vi "BLE v1.0.vi"(7 "Est Thresh Val":dbl, 8 "Threshold Value Analysis":bool, 9 "Model Name":string="and_RB_SSA", 10 "Ex_Mod_IDs":string[](array[string]), 11 "Sp_Id_Arr":string[](array[string])) -> (0 "Close 2":bool, 3 "Boolean  Expression":string)   [LabVIEW 2014]
uses:
  <vilib>/Utility/file.llb/Read From Spreadsheet File (DBL).vi
  <vilib>/Utility/file.llb/Read From Spreadsheet File (string).vi
panel:
  out "Input Status":bool
  out "% fitness":string
  out "Row header":string[](array[string])
  out "Simulation Data":string[][](table)
  in  "Close":bool
  out "No of I/ps":i32
  out "Thresh Val":dbl[](array[numeric])
  out "All Data":string[][](array[string])
  out "Analog Data":dbl[][](array[numeric])
  out "All Data":dbl[][](array[numeric])
  out "Index":i32[](array[numeric])
  out "C1_Ar":dbl[](array[numeric])
  out "C2_Ar":dbl[](array[numeric])
  out "C3_Ar":dbl[](array[numeric])
  out "C4_Ar":dbl[](array[numeric])
  out "Cs4_1s":i32
  out "Cs3_1s":i32
  out "Cs2_1s":i32
  out "Cs1_1s":i32
  out "var_4":i8
  out "var_3":i8
  out "var_2":i8
  out "var_1":i8
  out "case4":i32
  out "case3":i32
  out "case2":i32
  out "case1":i32
  out "C4":dbl
  out "C3":dbl
  out "C2":dbl
  out "C1":dbl
  out "Digital Data":bool[][](array[boolean])
  # "Logic Expression"
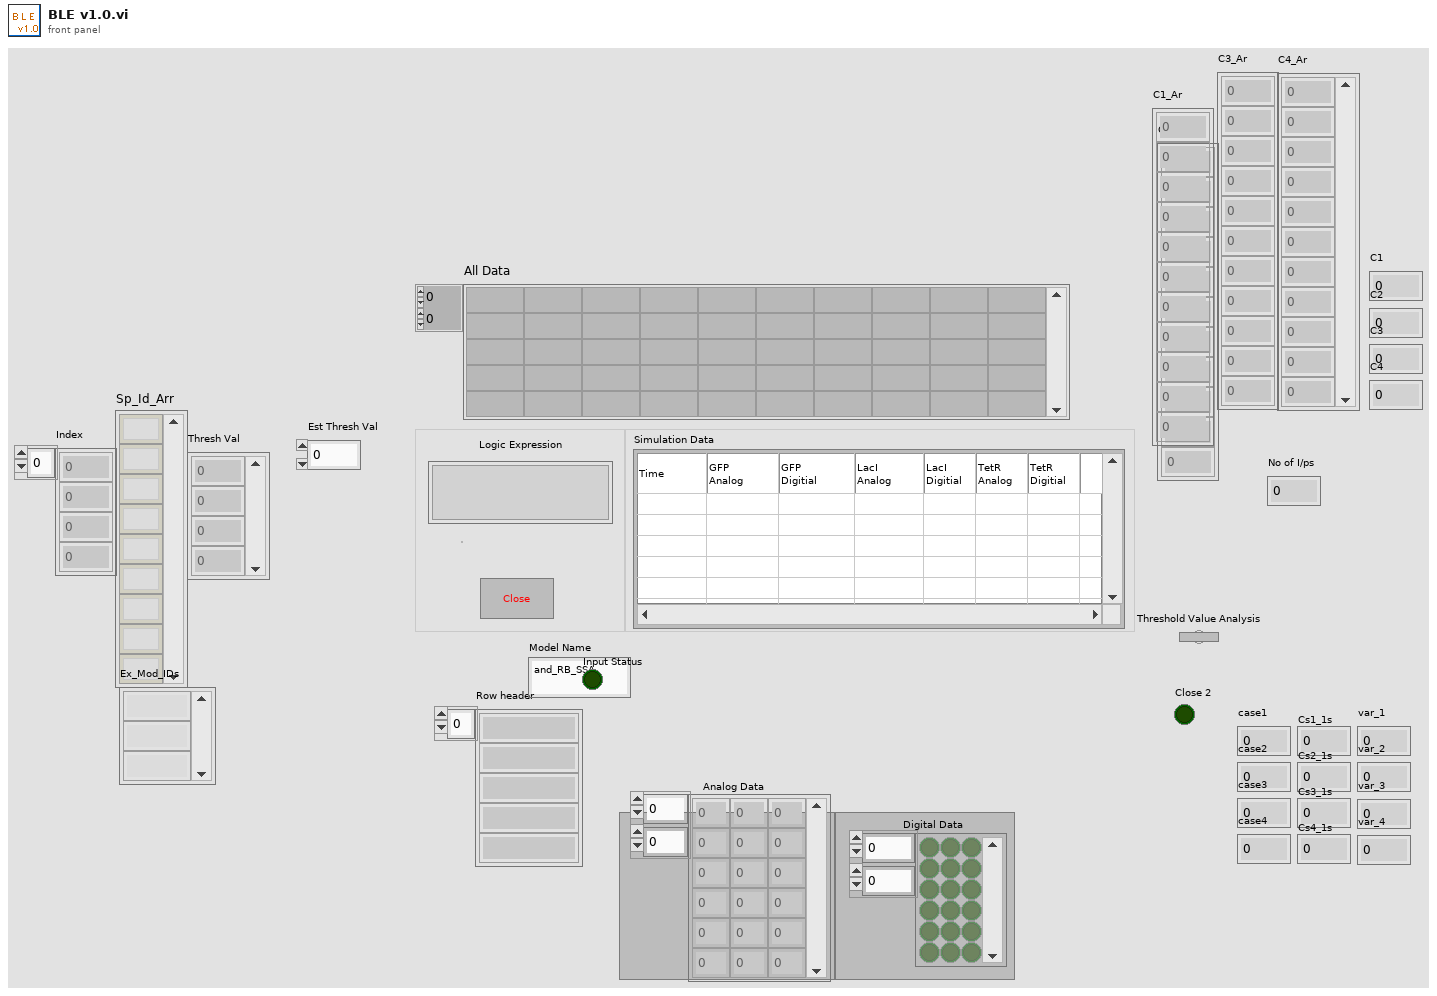
[diagram p1: front panel]
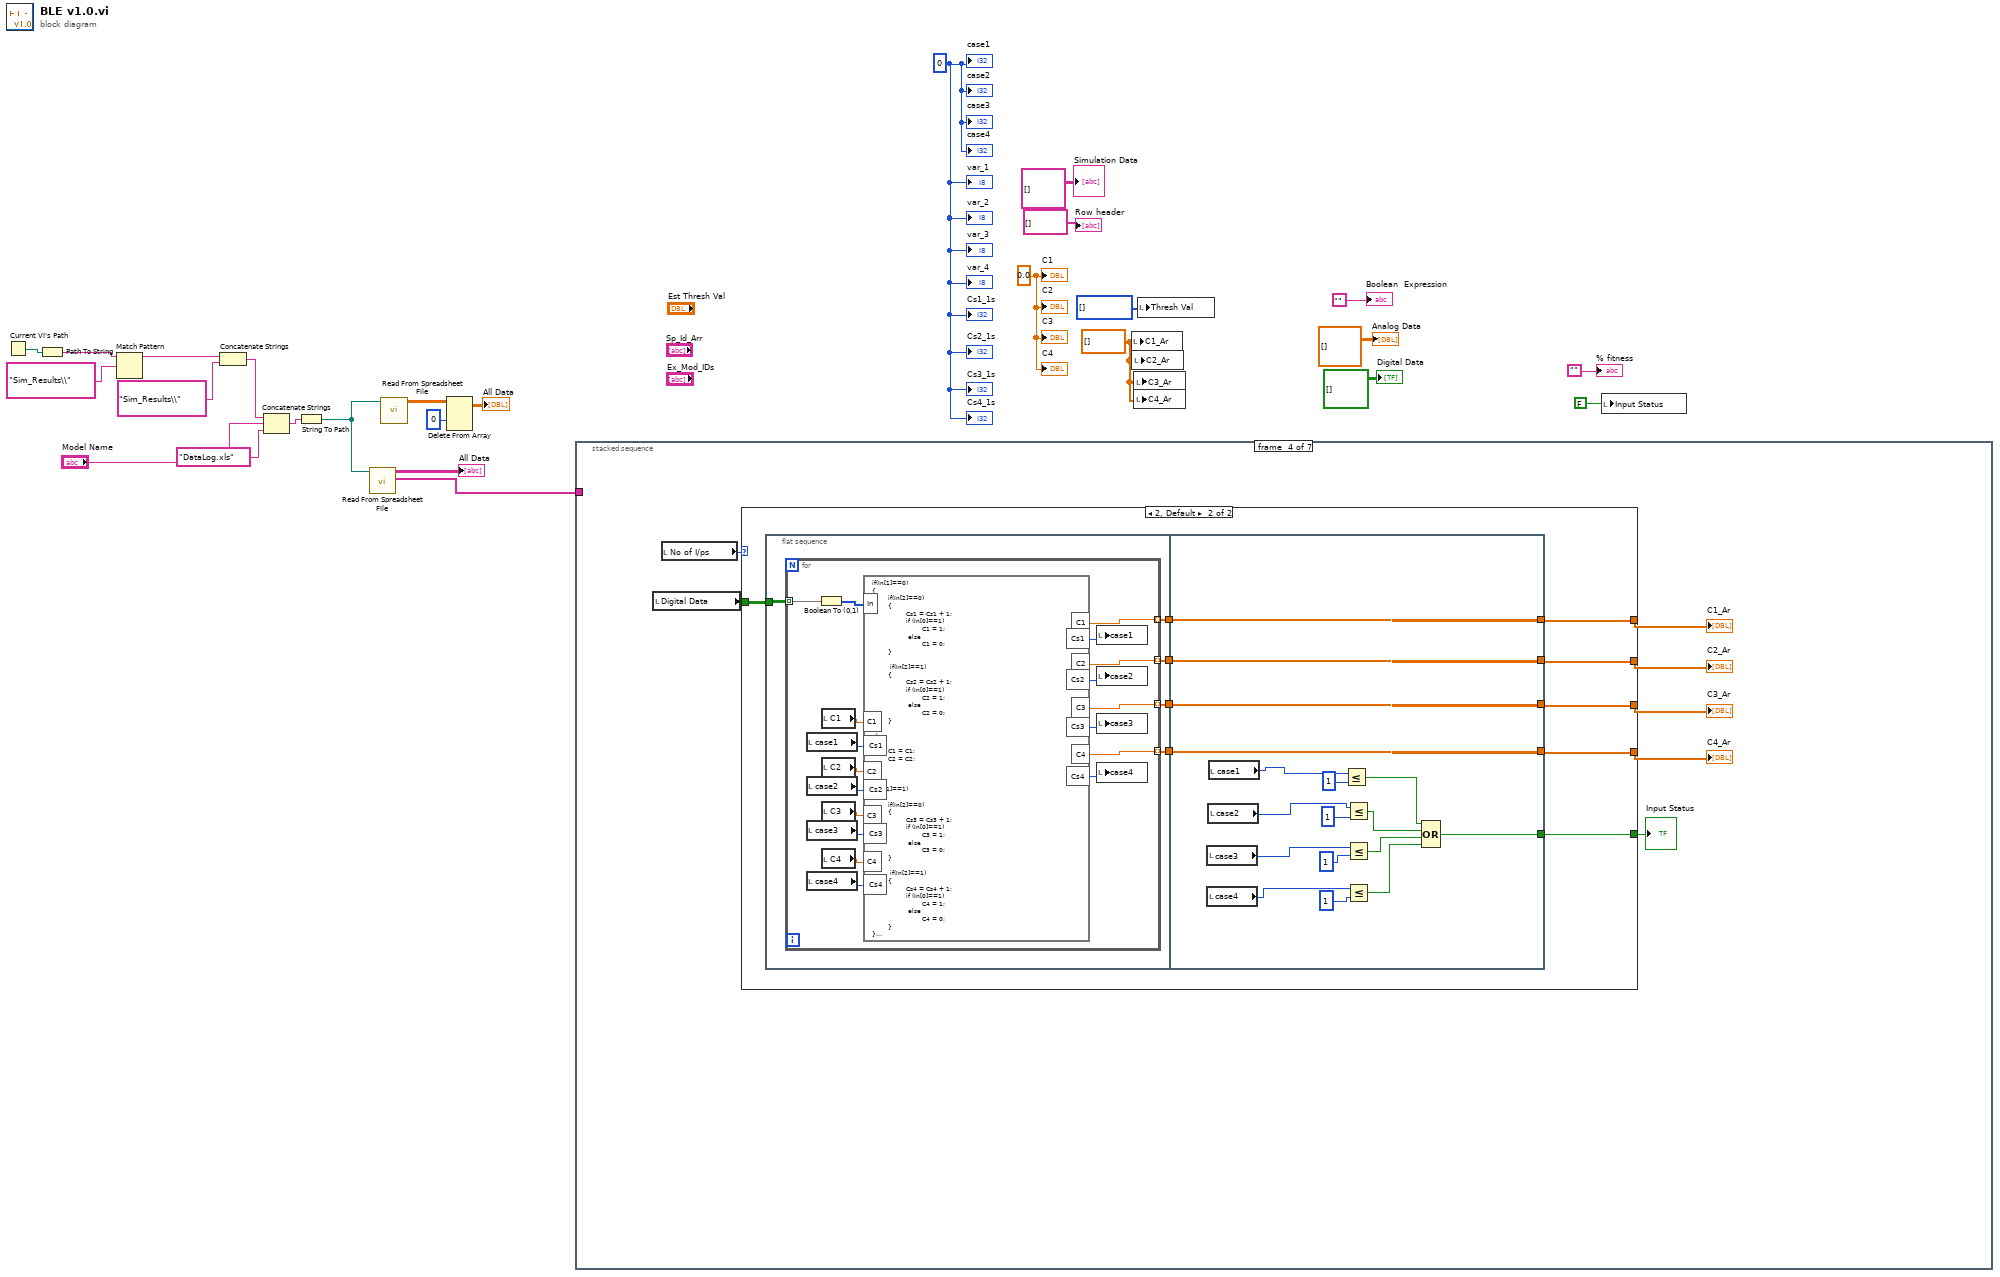
[diagram p0: block diagram]
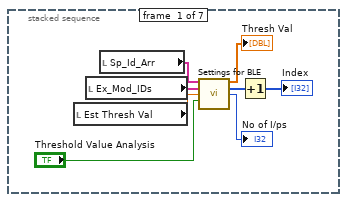
[diagram p2: hidden frame]
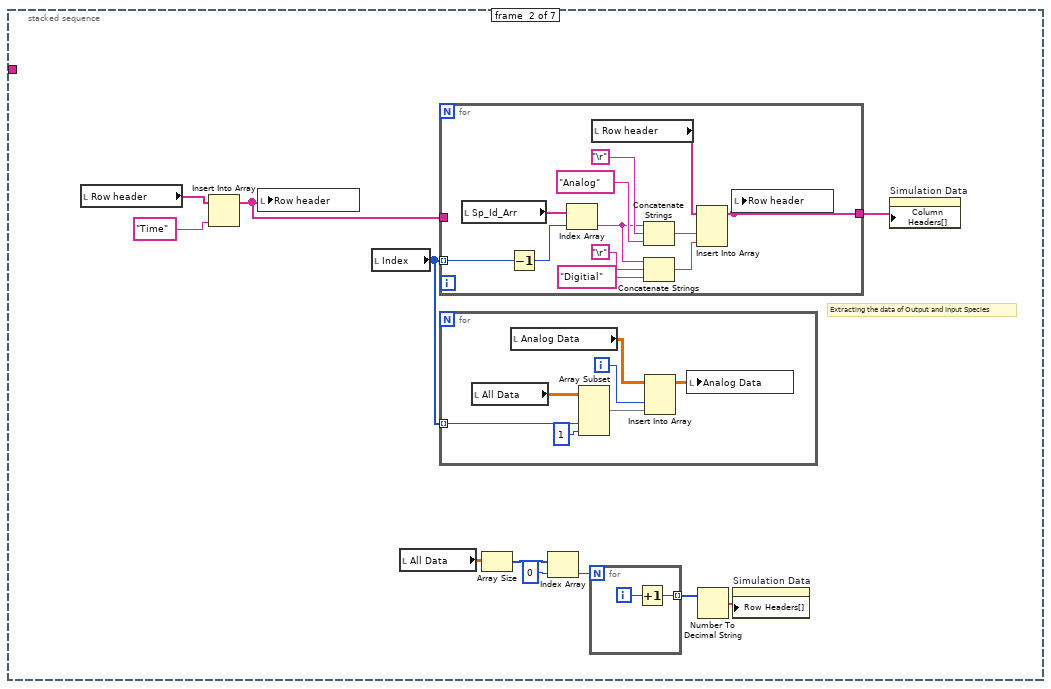
[diagram p3: hidden frame]
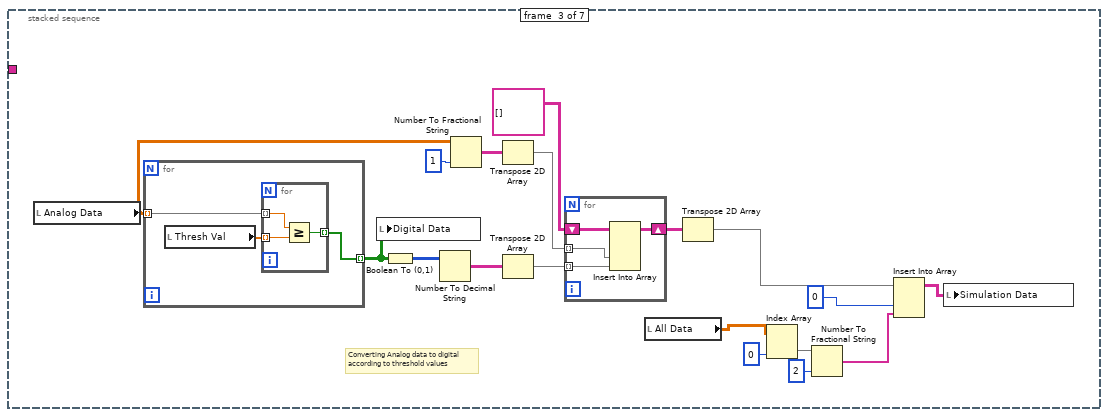
[diagram p4: hidden frame]
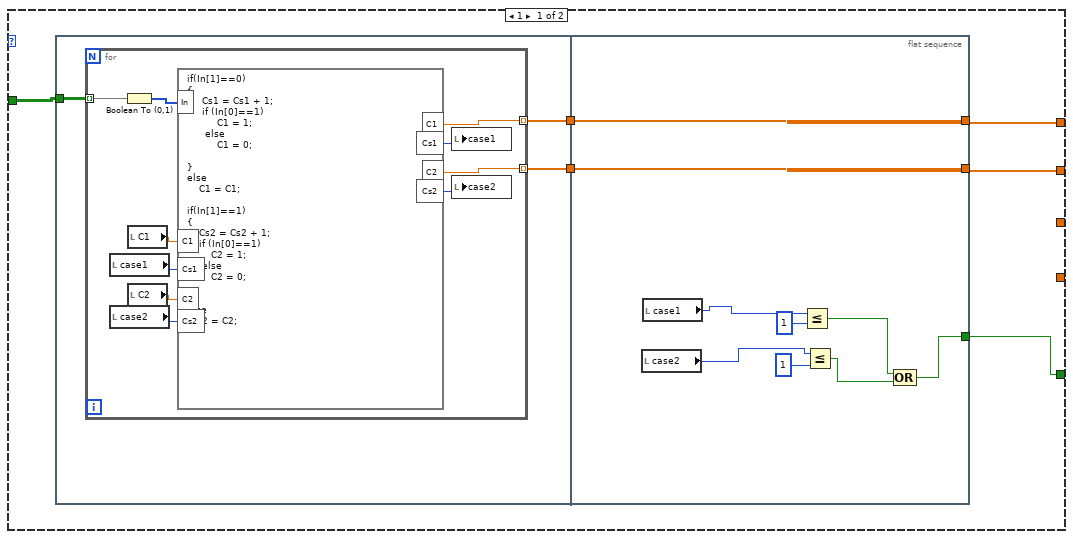
[diagram p5: hidden frame]
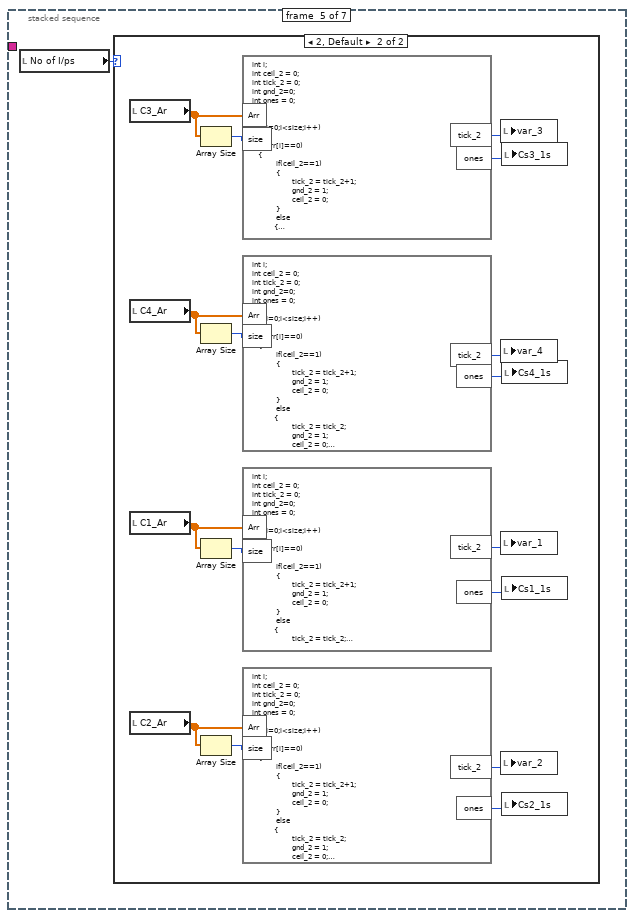
[diagram p6: hidden frame]
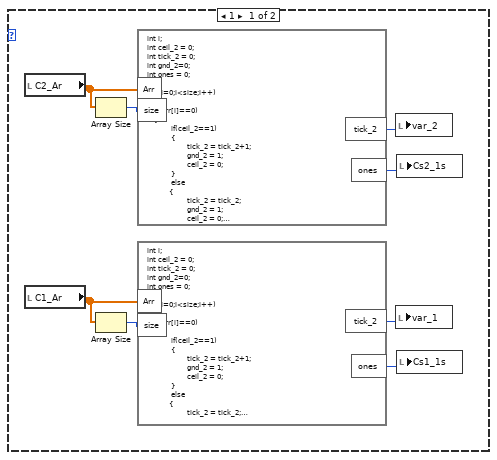
[diagram p7: hidden frame]
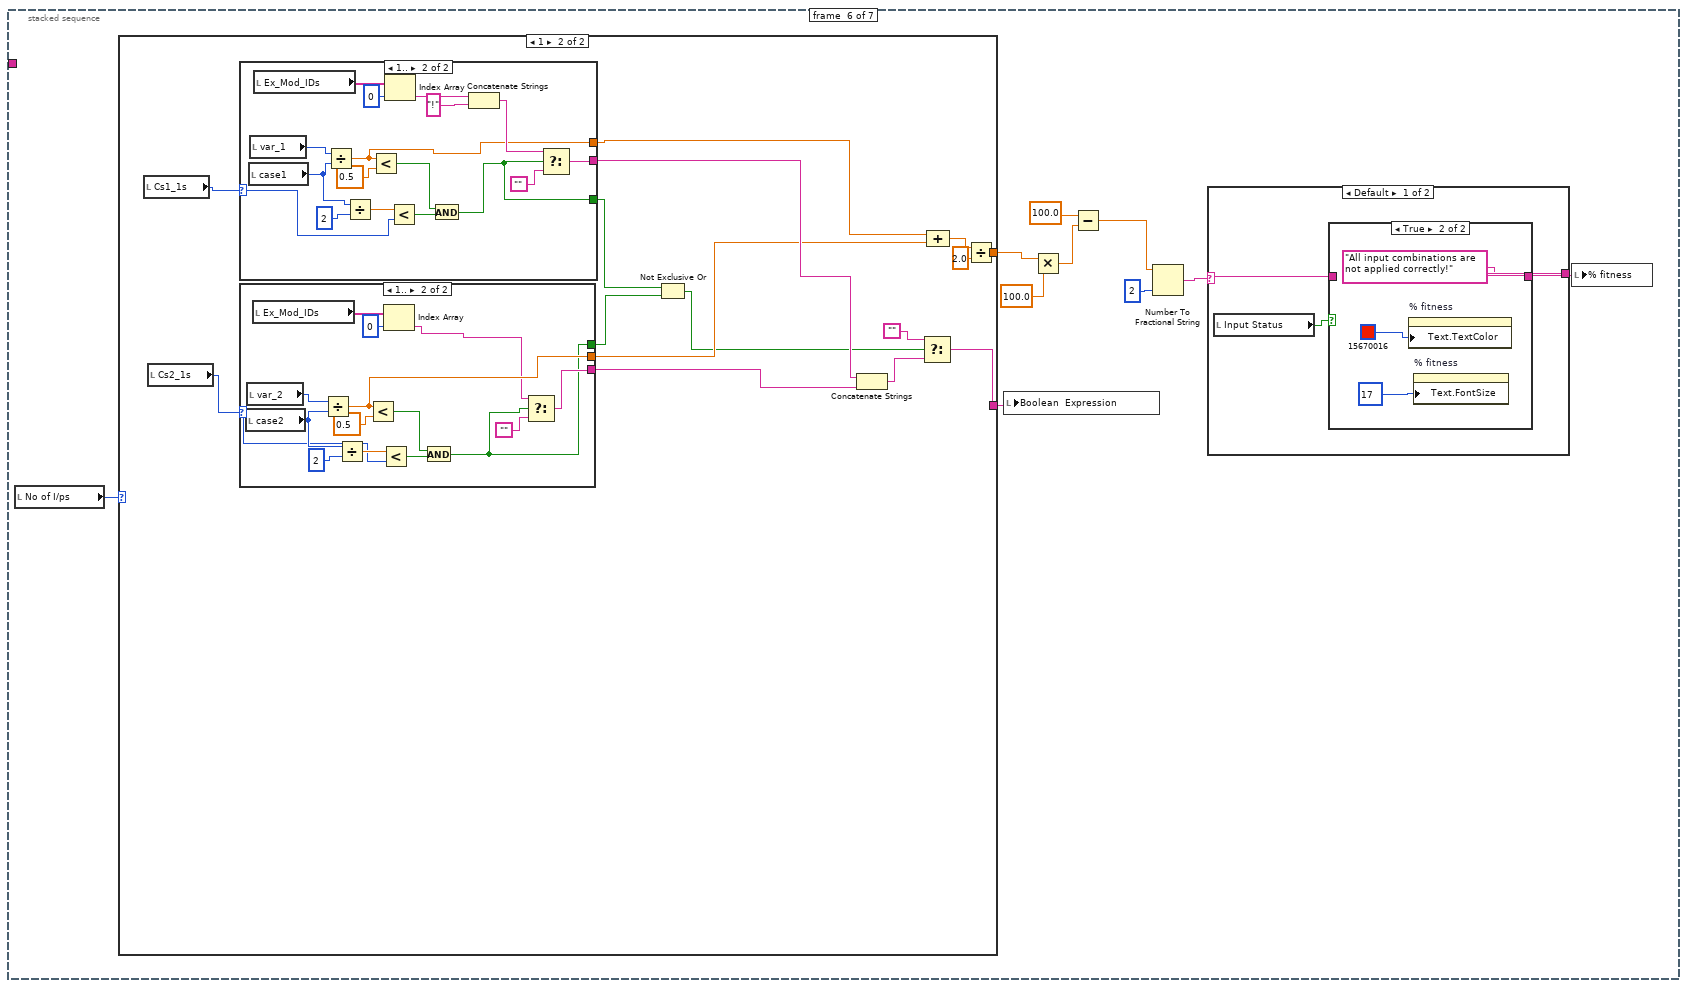
[diagram p8: hidden frame]
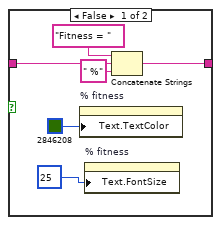
[diagram p9: hidden frame]
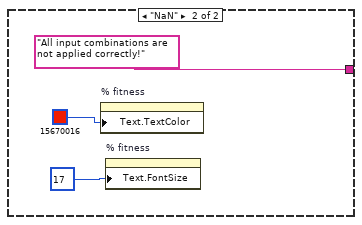
[diagram p10: hidden frame]
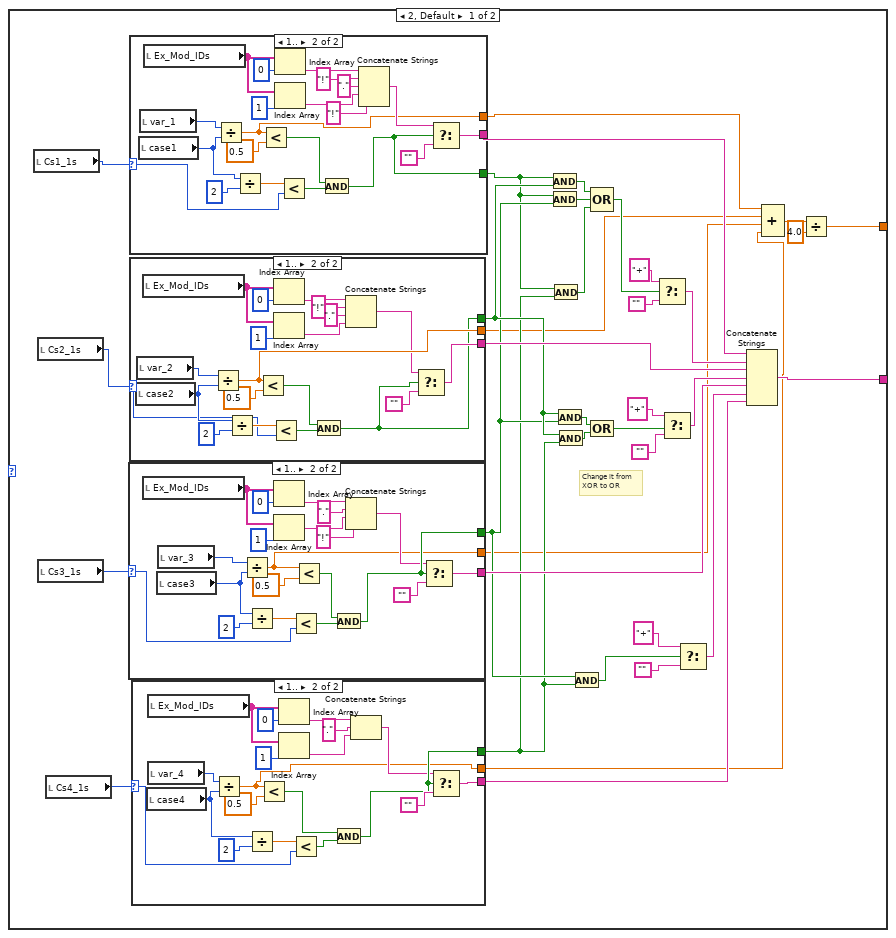
[diagram p11: hidden frame]
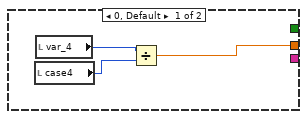
[diagram p12: hidden frame]
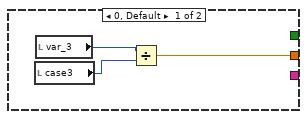
[diagram p13: hidden frame]
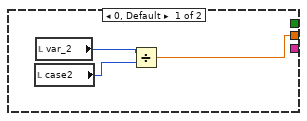
[diagram p14: hidden frame]
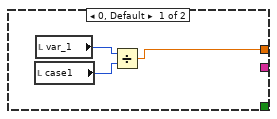
[diagram p15: hidden frame]
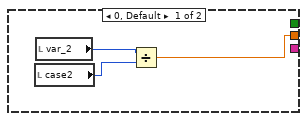
[diagram p16: hidden frame]
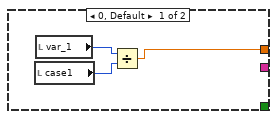
[diagram p17: hidden frame]
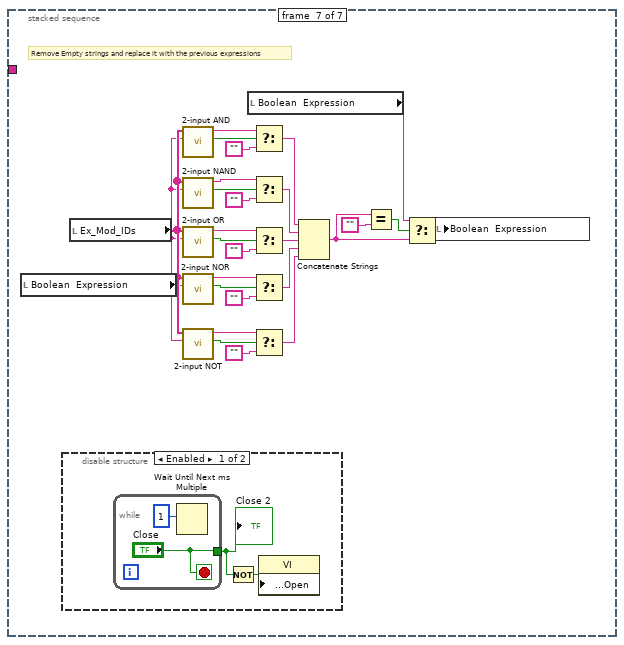
[diagram p18: hidden frame]
diagram:
  w21 = 0.0 ("C1")
  w22 = 0 ("case1")
  w26 = dbl[] [] ("C1_Ar")
  n1 = Current VI's Path() -> (path=w6:path)
  n2 = Path To String(path=w6) -> (string=w7:string)
  n3 = Match Pattern(string=w7, regular expression="Sim_Results\\" ("string")) -> (before substring=w9:string)  [unwired: 1 in, 3 out]
  n4 = Concatenate Strings(w9, "Sim_Results\\" ("string")) -> (w5:string)
  n5 = Concatenate Strings(w5, "Model Name", "DataLog.xls" ("name or relative path")) -> (w4:string)
  n6 = String To Path(string=w4) -> (path=w3:path)
  n7 = call-poly <vilib>:"Read From Spreadsheet File.vi"("file path (dialog if empty)"=w3) -> ("first row"=w13:string[], "all rows"=→"All Data":string[][])  [unwired: 6 in, 3 out]
  n8 = call-poly <vilib>:"Read From Spreadsheet File.vi"("file path (dialog if empty)"=w3) -> ("all rows"=w16:dbl[][])  [unwired: 6 in, 4 out]
  n9 = Delete From Array(array=w16, index (row)=0) -> (array with subset deleted=→"All Data":dbl[][])  [unwired: 2 in, 1 out]
  n10 = stacked-sequence {
    tunnel: w13 -> [_ _ _ _ _ _ _]
    frame #0 {
      n11 = local read "Est Thresh Val"() -> (w27:dbl)
      n12 = local read "Ex_Mod_IDs"() -> (w33:string[])
      n13 = local read "Sp_Id_Arr"() -> (w34:string[])
      n14 = call "Settings for BLE.vi"("Sp_Id_Arr"=w34, "Ex_Mod_IDs"=w33, "Est Thresh Val"=w27, "Threshold Value Analysis"="Threshold Value Analysis") -> ("Thresh Val"=→"Thresh Val":dbl[], "Index"=w31:i32[], "No of I/ps"=→"No of I/ps":i32)  [unwired: 9 in]
      n15 = Increment(x=w31) -> (x+1=→"Index":i32[])
    }
    frame #1 {
      # "Extracting the data of Output and Input Species"
      n16 = local read "Row header"() -> (w37:string[])
      n17 = Insert Into Array(array=w37, new element="Time" ("new element/subarray")) -> (w35:string[])  [unwired: 1 in]
      n18 = local write "Row header"(w35) -> ()
      n19 = local read "Index"() -> (w45:i32[])
      n20 = local read "All Data"() -> (w43:dbl[][])
      n21 = for {
        tunnel: w45 -> [w58] mode=indexing
        tunnel: [w49] -> w44
        tunnel: w35 -> [_]
        n22 = local read "Sp_Id_Arr"() -> (w59:string[])
        n23 = Decrement(x=w58) -> (x-1=w57:i32)
        n24 = Index Array(array=w59, index=w57) -> (element=w51:string)
        n25 = local read "Row header"() -> (w48:string[])
        n26 = Concatenate Strings(w51, "\r", "Analog" ("string")) -> (w54:string)
        n27 = Concatenate Strings(w51, "\r", "Digitial" ("string")) -> (w50:string)
        n28 = Insert Into Array(array=w48, new element #1=w54, new element #2=w50) -> (w49:string[])  [unwired: 1 in]
        n29 = local write "Row header"(w49) -> ()
      }
      n30 = for {
        tunnel: w45 -> [w65] mode=indexing
        i -> [w62]
        n31 = local read "All Data"() -> (w66:dbl[][])
        n32 = local read "Analog Data"() -> (w61:dbl[][])
        n33 = Array Subset(array=w66, index (col)=w65, length (col)=1 ("length")) -> (w63:dbl[][])  [unwired: 2 in]
        n34 = Insert Into Array(array=w61, index (col)=w62, new element=w63) -> (w60:dbl[][])  [unwired: 1 in]
        n35 = local write "Analog Data"(w60) -> ()
      }
      n36 = Array Size(array=w43) -> (size(s)=w42:i32[])
      n37 = Index Array(array=w42, index=0) -> (element=w40:i32)
      n38 = for {
        N: w40 -> [_]
        tunnel: [w46] -> w39 mode=indexing
        i -> [w47]
        n39 = Increment(x=w47) -> (x+1=w46:i32)
      }
      n40 = Number To Decimal String(number=w39) -> (decimal integer string=w38:string[])  [unwired: 1 in]
      n41 = property on="Simulation Data" class="Tbl (strict)"("Row Headers[]"=w38) -> ()  [unwired: 2 in, 2 out]
      n42 = property on="Simulation Data" class="Tbl (strict)"("Column Headers[]"=w44) -> ()  [unwired: 2 in, 2 out]
    }
    frame #2 {
      # "Converting Analog data to digital\naccording to threshold values"
      n43 = local read "Analog Data"() -> (w80:dbl[][])
      n44 = for {
        tunnel: w80 -> [w90] mode=indexing
        tunnel: [w89] -> w82 mode=indexing
        n45 = local read "Thresh Val"() -> (w91:dbl[])
        n46 = for {
          tunnel: w90 -> [w93] mode=indexing
          tunnel: w91 -> [w94] mode=indexing
          tunnel: [w92] -> w89 mode=indexing
          n47 = Greater Or Equal?(x=w93, y=w94) -> (x >= y?=w92:bool)
        }
      }
      n48 = local write "Digital Data"(w82) -> ()
      n49 = Boolean To (0,1)(Boolean=w82) -> (0, 1=w83:i16[][])
      n50 = Number To Decimal String(number=w83) -> (decimal integer string=w77:string[][])  [unwired: 1 in]
      n51 = Number To Fractional String(number=w80, precision (6)=i16 1) -> (F-format string=w79:string[][])  [unwired: 2 in]
      n52 = Transpose 2D Array(2D array=w79) -> (transposed array=w78:string[][])
      n53 = Transpose 2D Array(2D array=w77) -> (transposed array=w76:string[][])
      n54 = for {
        shift-right: [w88] -> w75
        shift-left: string[][] [] -> [w87]
        tunnel: w76 -> [w86] mode=indexing
        tunnel: w78 -> [w85] mode=indexing
        n55 = Insert Into Array(array=w87, new element #1=w85, new element #2=w86) -> (w88:string[][])  [unwired: 2 in]
      }
      n56 = local read "All Data"() -> (w68:dbl[][])
      n57 = Transpose 2D Array(2D array=w75) -> (transposed array=w69:string[][])
      n58 = Index Array(array=w68, index (col)=0 ("disabled index (col)")) -> (element=w71:dbl[])  [unwired: 1 in]
      n59 = Number To Fractional String(number=w71, precision (6)=i16 2) -> (F-format string=w73:string[])  [unwired: 2 in]
      n60 = Insert Into Array(array=w69, index (col)=0 ("disabled index (col)"), new element=w73) -> (w67:string[][])  [unwired: 1 in]
      n61 = local write "Simulation Data"(w67) -> ()
    }
    frame #3 {
      n62 = local read "Digital Data"() -> (w101:bool[][])
      n63 = local read "No of I/ps"() -> (w96:i32)
      n64 = case shown="2, Default" w96 {
        tunnel: w101 -> [w107 w139]
        tunnel: [w105 w138] -> w100
        tunnel: [w106 w137] -> w99
        tunnel: [_ w136] -> w98
        tunnel: [_ w135] -> w97
        tunnel: [w102 w130] -> w95
        frame 1 {
          n65 = flat-sequence {
            tunnel: w107 -> [w110]
            tunnel: [w109] -> w104
            tunnel: [w108] -> w103
            tunnel: [w128] -> w105
            tunnel: [w129] -> w106
            tunnel: w104 -> [w129]
            tunnel: w103 -> [w128]
            tunnel: [w121] -> w102
            frame #0 {
              n66 = for {
                tunnel: [w113] -> w108 mode=indexing
                tunnel: [w112] -> w109 mode=indexing
                tunnel: w110 -> [w111] mode=indexing
                n67 = local read "case1"() -> (w118:i32)
                n68 = local read "case2"() -> (w117:i32)
                n69 = Boolean To (0,1)(Boolean=w111) -> (0, 1=w120:i16[])
                n70 = local read "C1"() -> (w116:dbl)
                n71 = local read "C2"() -> (w119:dbl)
                n72 = formula code="if(In[1]==0)\n{\n     Cs1 = Cs1 + 1;\n     if (In[0]==1)\n          C1 = 1;\n      else\n          C1 = 0;\n\n}\nelse\n    C1 = C1;\n\nif(In[1]==1)\n{\n    Cs2 = Cs2 + 1;\n    if (In[0]==1)\n        C2 = 1;\n     else\n        C2 = 0;\n\n}\nelse\n   C2 = C2;"("In"=w120, "C1"=w116, "C2"=w119, "Cs1"=w118, "Cs2"=w117) -> ("C1"=w113:dbl, "C2"=w112:dbl, "Cs1"=w114:i32, "Cs2"=w115:i32)
                n73 = local write "case1"(w114) -> ()
                n74 = local write "case2"(w115) -> ()
              }
            }
            frame #1 {
              n75 = local read "case2"() -> (w122:i32)
              n76 = local read "case1"() -> (w123:i32)
              n77 = Less Or Equal?(x=w123, y=1) -> (x <= y?=w125:bool)
              n78 = Less Or Equal?(x=w122, y=1) -> (x <= y?=w124:bool)
              n79 = Compound Arithmetic op=OR(w125, w124) -> (w121:bool)
            }
          }
        }
        frame 2, Default {
          n80 = flat-sequence {
            tunnel: w139 -> [w144]
            tunnel: [w143] -> w134
            tunnel: [w142] -> w133
            tunnel: [w141] -> w132
            tunnel: [w140] -> w131
            tunnel: [w176] -> w135
            tunnel: [w177] -> w136
            tunnel: [w178] -> w137
            tunnel: [w179] -> w138
            tunnel: w134 -> [w179]
            tunnel: w133 -> [w178]
            tunnel: w132 -> [w177]
            tunnel: w131 -> [w176]
            tunnel: [w163] -> w130
            frame #0 {
              n81 = for {
                tunnel: w144 -> [w162] mode=indexing
                tunnel: [w148] -> w143 mode=indexing
                tunnel: [w147] -> w142 mode=indexing
                tunnel: [w146] -> w141 mode=indexing
                tunnel: [w145] -> w140 mode=indexing
                n82 = local read "case1"() -> (w157:i32)
                n83 = local read "case2"() -> (w154:i32)
                n84 = local read "case3"() -> (w156:i32)
                n85 = local read "case4"() -> (w155:i32)
                n86 = Boolean To (0,1)(Boolean=w162) -> (0, 1=w161:i16[])
                n87 = local read "C1"() -> (w153:dbl)
                n88 = local read "C2"() -> (w160:dbl)
                n89 = local read "C3"() -> (w159:dbl)
                n90 = local read "C4"() -> (w158:dbl)
                n91 = formula code="if(In[1]==0)\n{\n        if(In[2]==0)\n        {\n                 Cs1 = Cs1 + 1;\n                 if (In[0]==1)\n                         C1 = 1;\n                  else\n                         C1 = 0;\n        }\n\n         if(In[2]==1)\n        {\n                 Cs2 = Cs2 + 1;\n                 if (In[0]==1)\n                         C2 = 1;\n                  else\n                         C2 = 0;\n        }  \n}\nelse\n{\n        C1 = C1;\n        C2 = C2;\n}\n\n\nif(In[1]==1)\n{\n        if(In[2]==0)\n        {\n                 Cs3 = Cs3 + 1;\n                 if (In[0]==1)\n                         C3 = 1;\n                  else\n                         C3 = 0;\n        }\n\n         if(In[2]==1)\n        {\n                 Cs4 = Cs4 + 1;\n                 if (In[0]==1)\n                         C4 = 1;\n                  else\n                         C4 = 0;\n        }  \n}\nelse\n{\n        C3 = C3;\n        C4 = C4;\n}"("In"=w161, "C1"=w153, "C2"=w160, "C3"=w159, "C4"=w158, "Cs1"=w157, "Cs2"=w154, "Cs3"=w156, "Cs4"=w155) -> ("C1"=w148:dbl, "C2"=w147:dbl, "C3"=w146:dbl, "C4"=w145:dbl, "Cs1"=w149:i32, "Cs2"=w150:i32, "Cs3"=w151:i32, "Cs4"=w152:i32)
                n92 = local write "case1"(w149) -> ()
                n93 = local write "case2"(w150) -> ()
                n94 = local write "case3"(w151) -> ()
                n95 = local write "case4"(w152) -> ()
              }
            }
            frame #1 {
              n96 = local read "case3"() -> (w165:i32)
              n97 = local read "case4"() -> (w164:i32)
              n98 = local read "case2"() -> (w166:i32)
              n99 = local read "case1"() -> (w167:i32)
              n100 = Less Or Equal?(x=w167, y=1) -> (x <= y?=w171:bool)
              n101 = Less Or Equal?(x=w166, y=1) -> (x <= y?=w170:bool)
              n102 = Less Or Equal?(x=w165, y=1) -> (x <= y?=w169:bool)
              n103 = Less Or Equal?(x=w164, y=1) -> (x <= y?=w168:bool)
              n104 = Compound Arithmetic op=OR(w171, w170, w169, w168) -> (w163:bool)
            }
          }
        }
      }
      "C1_Ar" <- w100
      "C2_Ar" <- w99
      "C3_Ar" <- w98
      "C4_Ar" <- w97
      "Input Status" <- w95
    }
    frame #4 {
      n105 = local read "No of I/ps"() -> (w180:i32)
      n106 = case shown="2, Default" w180 {
        frame 1 {
          n107 = local read "C2_Ar"() -> (w185:dbl[])
          n108 = local read "C1_Ar"() -> (w186:dbl[])
          n109 = Array Size(array=w185) -> (size(s)=w187:i32)
          n110 = Array Size(array=w186) -> (size(s)=w188:i32)
          n111 = formula code="int i;\nint ceil_2 = 0;\nint tick_2 = 0;\nint gnd_2=0;\nint ones = 0;\n\nfor (i=0;i<size;i++)\n{\n   if(Arr[i]==0)\n   { \n            if(ceil_2==1)\n            {\n                    tick_2 = tick_2+1;\n                    gnd_2 = 1;\n                    ceil_2 = 0;\n            }\n            else \n           {\n                    tick_2 = tick_2;\n                    gnd_2 = 1;\n                    ceil_2 = 0;                 \n           } \n   }\n   \n   else if(Arr[i]==1)\n   {\n            ones = ones +1;\n            if(gnd_2==1)\n            {\n                    tick_2 = tick_2+1;\n                    gnd_2 = 0;\n                    ceil_2 = 1;\n            }\n            else \n           {\n                    tick_2 = tick_2;\n                    gnd_2 = gnd_2;\n                    ceil_2 = 1;                 \n           } \n   }\n   else\n   {\n           tick_2 = tick_2;\n           ceil_2 = ceil_2;\n           gnd_2 = gnd_2;\n   }\n}"("Arr"=w185, "size"=w187) -> ("tick_2"=w182:i32, "ones"=w181:i32)
          n112 = formula code="int i;\nint ceil_2 = 0;\nint tick_2 = 0;\nint gnd_2=0;\nint ones = 0;\n\nfor (i=0;i<size;i++)\n{\n   if(Arr[i]==0)\n   { \n            if(ceil_2==1)\n            {\n                    tick_2 = tick_2+1;\n                    gnd_2 = 1;\n                    ceil_2 = 0;\n            }\n            else \n           {\n                    tick_2 = tick_2;\n                    gnd_2 = 1;\n                    ceil_2 = 0;                 \n           } \n   }\n   \n   else if(Arr[i]==1)\n   {\n            ones = ones +1;\n            if(gnd_2==1)\n            {\n                    tick_2 = tick_2+1;\n                    gnd_2 = 0;\n                    ceil_2 = 1;\n            }\n            else \n           {\n                    tick_2 = tick_2;\n                    gnd_2 = gnd_2;\n                    ceil_2 = 1;                 \n           } \n   }\n   else\n   {\n           tick_2 = tick_2;\n           ceil_2 = ceil_2;\n           gnd_2 = gnd_2;\n   }\n}"("Arr"=w186, "size"=w188) -> ("tick_2"=w184:i32, "ones"=w183:i32)
          n113 = local write "var_2"(w182) -> ()
          n114 = local write "var_1"(w184) -> ()
          n115 = local write "Cs2_1s"(w181) -> ()
          n116 = local write "Cs1_1s"(w183) -> ()
        }
        frame 2, Default {
          n117 = local read "C3_Ar"() -> (w197:dbl[])
          n118 = local read "C4_Ar"() -> (w199:dbl[])
          n119 = local read "C1_Ar"() -> (w200:dbl[])
          n120 = local read "C2_Ar"() -> (w198:dbl[])
          n121 = Array Size(array=w197) -> (size(s)=w203:i32)
          n122 = Array Size(array=w199) -> (size(s)=w201:i32)
          n123 = Array Size(array=w200) -> (size(s)=w204:i32)
          n124 = Array Size(array=w198) -> (size(s)=w202:i32)
          n125 = formula code="int i;\nint ceil_2 = 0;\nint tick_2 = 0;\nint gnd_2=0;\nint ones = 0;\n\n\nfor (i=0;i<size;i++)\n{\n   if(Arr[i]==0)\n   { \n            if(ceil_2==1)\n            {\n                    tick_2 = tick_2+1;\n                    gnd_2 = 1;\n                    ceil_2 = 0;\n            }\n            else \n           {\n                    tick_2 = tick_2;\n                    gnd_2 = 1;\n                    ceil_2 = 0;                 \n           } \n   }\n   \n   else if(Arr[i]==1)\n   {\n            ones = ones +1;\n            if(gnd_2==1)\n            {\n                    tick_2 = tick_2+1;\n                    gnd_2 = 0;\n                    ceil_2 = 1;\n            }\n            else \n           {\n                    tick_2 = tick_2;\n                    gnd_2 = gnd_2;\n                    ceil_2 = 1;                 \n           } \n   }\n   else\n   {\n           tick_2 = tick_2;\n           ceil_2 = ceil_2;\n           gnd_2 = gnd_2;\n   }\n}"("Arr"=w197, "size"=w203) -> ("tick_2"=w192:i32, "ones"=w191:i32)
          n126 = formula code="int i;\nint ceil_2 = 0;\nint tick_2 = 0;\nint gnd_2=0;\nint ones = 0;\n\nfor (i=0;i<size;i++)\n{\n   if(Arr[i]==0)\n   { \n            if(ceil_2==1)\n            {\n                    tick_2 = tick_2+1;\n                    gnd_2 = 1;\n                    ceil_2 = 0;\n            }\n            else \n           {\n                    tick_2 = tick_2;\n                    gnd_2 = 1;\n                    ceil_2 = 0;                 \n           } \n   }\n   \n   else if(Arr[i]==1)\n   {\n            ones = ones +1;\n            if(gnd_2==1)\n            {\n                    tick_2 = tick_2+1;\n                    gnd_2 = 0;\n                    ceil_2 = 1;\n            }\n            else \n           {\n                    tick_2 = tick_2;\n                    gnd_2 = gnd_2;\n                    ceil_2 = 1;                 \n           } \n   }\n   else\n   {\n           tick_2 = tick_2;\n           ceil_2 = ceil_2;\n           gnd_2 = gnd_2;\n   }\n}"("Arr"=w199, "size"=w201) -> ("tick_2"=w190:i32, "ones"=w189:i32)
          n127 = formula code="int i;\nint ceil_2 = 0;\nint tick_2 = 0;\nint gnd_2=0;\nint ones = 0;\n\nfor (i=0;i<size;i++)\n{\n   if(Arr[i]==0)\n   { \n            if(ceil_2==1)\n            {\n                    tick_2 = tick_2+1;\n                    gnd_2 = 1;\n                    ceil_2 = 0;\n            }\n            else \n           {\n                    tick_2 = tick_2;\n                    gnd_2 = 1;\n                    ceil_2 = 0;                 \n           } \n   }\n   \n   else if(Arr[i]==1)\n   {\n            ones = ones +1;\n            if(gnd_2==1)\n            {\n                    tick_2 = tick_2+1;\n                    gnd_2 = 0;\n                    ceil_2 = 1;\n            }\n            else \n           {\n                    tick_2 = tick_2;\n                    gnd_2 = gnd_2;\n                    ceil_2 = 1;                 \n           } \n   }\n   else\n   {\n           tick_2 = tick_2;\n           ceil_2 = ceil_2;\n           gnd_2 = gnd_2;\n   }\n}"("Arr"=w200, "size"=w204) -> ("tick_2"=w196:i32, "ones"=w195:i32)
          n128 = formula code="int i;\nint ceil_2 = 0;\nint tick_2 = 0;\nint gnd_2=0;\nint ones = 0;\n\nfor (i=0;i<size;i++)\n{\n   if(Arr[i]==0)\n   { \n            if(ceil_2==1)\n            {\n                    tick_2 = tick_2+1;\n                    gnd_2 = 1;\n                    ceil_2 = 0;\n            }\n            else \n           {\n                    tick_2 = tick_2;\n                    gnd_2 = 1;\n                    ceil_2 = 0;                 \n           } \n   }\n   \n   else if(Arr[i]==1)\n   {\n            ones = ones +1;\n            if(gnd_2==1)\n            {\n                    tick_2 = tick_2+1;\n                    gnd_2 = 0;\n                    ceil_2 = 1;\n            }\n            else \n           {\n                    tick_2 = tick_2;\n                    gnd_2 = gnd_2;\n                    ceil_2 = 1;                 \n           } \n   }\n   else\n   {\n           tick_2 = tick_2;\n           ceil_2 = ceil_2;\n           gnd_2 = gnd_2;\n   }\n}"("Arr"=w198, "size"=w202) -> ("tick_2"=w194:i32, "ones"=w193:i32)
          n129 = local write "var_3"(w192) -> ()
          n130 = local write "var_4"(w190) -> ()
          n131 = local write "var_1"(w196) -> ()
          n132 = local write "var_2"(w194) -> ()
          n133 = local write "Cs3_1s"(w191) -> ()
          n134 = local write "Cs4_1s"(w189) -> ()
          n135 = local write "Cs1_1s"(w195) -> ()
          n136 = local write "Cs2_1s"(w193) -> ()
        }
      }
    }
    frame #5 {
      n137 = local read "No of I/ps"() -> (w211:i32)
      n138 = case shown="1" w211 {
        tunnel: [w249 w359] -> w214
        tunnel: [w230 w363] -> w212
        frame 2, Default {
          # "Change it from\nXOR to OR"
          n139 = local read "Cs1_1s"() -> (w266:i32)
          n140 = local read "Cs2_1s"() -> (w265:i32)
          n141 = local read "Cs3_1s"() -> (w264:i32)
          n142 = local read "Cs4_1s"() -> (w263:i32)
          n143 = case shown="1.." w264 {
            selector: w264 -> [_ w303]
            tunnel: [_ w301] -> w240
            tunnel: [_ w308] -> w252
            tunnel: [w289 w292] -> w234
            frame 0, Default {
              n144 = local read "case3"() -> (w291:i32)
              n145 = local read "var_3"() -> (w290:i8)
              n146 = Divide(x=w290, y=w291) -> (x/y=w289:dbl)
            }
            frame 1.. {
              n147 = local read "Ex_Mod_IDs"() -> (w295:string[])
              n148 = local read "case3"() -> (w304:i32)
              n149 = local read "var_3"() -> (w309:i8)
              n150 = Divide(x=w309, y=w304) -> (x/y=w292:dbl)
              n151 = Divide(x=w304, y=i8 2) -> (x/y=w307:dbl)
              n152 = Index Array(array=w295, index=0) -> (element=w298:string)
              n153 = Index Array(array=w295, index=1) -> (element=w296:string)
              n154 = Less?(x=w307, y=w303) -> (x < y?=w305:bool)
              n155 = Less?(x=w292, y=0.5) -> (x < y?=w302:bool)
              n156 = And(x=w302, y=w305) -> (x .and. y?=w301:bool)
              n157 = Concatenate Strings(w298, "." ("string"), w296, "!" ("string")) -> (w293:string)
              n158 = Select(t=w293, s=w301, f="") -> (s? t:f=w308:string)
            }
          }
          n159 = case shown="1.." w266 {
            selector: w266 -> [_ w350]
            tunnel: [_ w348] -> w237
            tunnel: [_ w355] -> w256
            tunnel: [w335 w338] -> w236
            frame 0, Default {
              n160 = local read "case1"() -> (w337:i32)
              n161 = local read "var_1"() -> (w336:i8)
              n162 = Divide(x=w336, y=w337) -> (x/y=w335:dbl)
            }
            frame 1.. {
              n163 = local read "case1"() -> (w351:i32)
              n164 = local read "var_1"() -> (w356:i8)
              n165 = local read "Ex_Mod_IDs"() -> (w339:string[])
              n166 = Divide(x=w356, y=w351) -> (x/y=w338:dbl)
              n167 = Divide(x=w351, y=i8 2) -> (x/y=w354:dbl)
              n168 = Less?(x=w338, y=0.5) -> (x < y?=w349:bool)
              n169 = Index Array(array=w339, index=0) -> (element=w345:string)
              n170 = Index Array(array=w339, index=1) -> (element=w342:string)
              n171 = Less?(x=w354, y=w350) -> (x < y?=w352:bool)
              n172 = And(x=w349, y=w352) -> (x .and. y?=w348:bool)
              n173 = Concatenate Strings(w345, "!" ("t"), "." ("string"), w342, "!" ("t")) -> (w340:string)
              n174 = Select(t=w340, s=w348, f="") -> (s? t:f=w355:string)
            }
          }
          n175 = case shown="1.." w265 {
            selector: w265 -> [_ w325]
            tunnel: [_ w323] -> w244
            tunnel: [_ w331] -> w254
            tunnel: [w312 w330] -> w235
            frame 0, Default {
              n176 = local read "case2"() -> (w313:i32)
              n177 = local read "var_2"() -> (w314:i8)
              n178 = Divide(x=w314, y=w313) -> (x/y=w312:dbl)
            }
            frame 1.. {
              n179 = local read "case2"() -> (w326:i32)
              n180 = local read "var_2"() -> (w332:i8)
              n181 = local read "Ex_Mod_IDs"() -> (w322:string[])
              n182 = Divide(x=w332, y=w326) -> (x/y=w330:dbl)
              n183 = Divide(x=w326, y=i8 2) -> (x/y=w327:dbl)
              n184 = Less?(x=w330, y=0.5) -> (x < y?=w324:bool)
              n185 = Less?(x=w327, y=w325) -> (x < y?=w329:bool)
              n186 = Index Array(array=w322, index=0) -> (element=w318:string)
              n187 = Index Array(array=w322, index=1) -> (element=w321:string)
              n188 = And(x=w324, y=w329) -> (x .and. y?=w323:bool)
              n189 = Concatenate Strings(w318, "!" ("t"), "." ("string"), w321) -> (w315:string)
              n190 = Select(t=w315, s=w323, f="") -> (s? t:f=w331:string)
            }
          }
          n191 = case shown="1.." w263 {
            selector: w263 -> [_ w281]
            tunnel: [_ w278] -> w239
            tunnel: [_ w285] -> w250
            tunnel: [w267 w270] -> w233
            frame 0, Default {
              n192 = local read "case4"() -> (w268:i32)
              n193 = local read "var_4"() -> (w269:i8)
              n194 = Divide(x=w269, y=w268) -> (x/y=w267:dbl)
            }
            frame 1.. {
              n195 = local read "case4"() -> (w280:i32)
              n196 = local read "Ex_Mod_IDs"() -> (w277:string[])
              n197 = local read "var_4"() -> (w286:i8)
              n198 = Divide(x=w286, y=w280) -> (x/y=w270:dbl)
              n199 = Divide(x=w280, y=i8 2) -> (x/y=w282:dbl)
              n200 = Less?(x=w270, y=0.5) -> (x < y?=w279:bool)
              n201 = Index Array(array=w277, index=0) -> (element=w274:string)
              n202 = Index Array(array=w277, index=1) -> (element=w276:string)
              n203 = Less?(x=w282, y=w281) -> (x < y?=w284:bool)
              n204 = And(x=w279, y=w284) -> (x .and. y?=w278:bool)
              n205 = Concatenate Strings(w274, "." ("string"), w276) -> (w271:string)
              n206 = Select(t=w271, s=w278, f="") -> (s? t:f=w285:string)
            }
          }
          n207 = And(x=w237, y=w244) -> (x .and. y?=w247:bool)
          n208 = And(x=w237, y=w240) -> (x .and. y?=w246:bool)
          n209 = And(x=w237, y=w239) -> (x .and. y?=w245:bool)
          n210 = And(x=w244, y=w240) -> (x .and. y?=w242:bool)
          n211 = And(x=w244, y=w239) -> (x .and. y?=w241:bool)
          n212 = And(x=w240, y=w239) -> (x .and. y?=w238:bool)
          n213 = Compound Arithmetic op=OR(w247, w246, w245) -> (w248:bool)
          n214 = Compound Arithmetic op=OR(w242, w241) -> (w243:bool)
          n215 = Select(t="+", s=w248, f="") -> (s? t:f=w255:string)
          n216 = Select(t="+", s=w243, f="") -> (s? t:f=w253:string)
          n217 = Select(t="+", s=w238, f="") -> (s? t:f=w251:string)
          n218 = Concatenate Strings(w256, w255, w254, w253, w252, w251, w250) -> (w249:string)
          n219 = Compound Arithmetic op=ADD(w236, w235, w234, w233) -> (w231:dbl)
          n220 = Divide(x=w231, y=4.0) -> (x/y=w230:dbl)
        }
        frame 1 {
          n221 = local read "Cs1_1s"() -> (w373:i32)
          n222 = local read "Cs2_1s"() -> (w372:i32)
          n223 = case shown="1.." w373 {
            selector: w373 -> [_ w403]
            tunnel: [_ w401] -> w368
            tunnel: [_ w408] -> w371
            tunnel: [w392 w395] -> w367
            frame 0, Default {
              n224 = local read "case1"() -> (w394:i32)
              n225 = local read "var_1"() -> (w393:i8)
              n226 = Divide(x=w393, y=w394) -> (x/y=w392:dbl)
            }
            frame 1.. {
              n227 = local read "case1"() -> (w404:i32)
              n228 = local read "var_1"() -> (w409:i8)
              n229 = local read "Ex_Mod_IDs"() -> (w396:string[])
              n230 = Divide(x=w409, y=w404) -> (x/y=w395:dbl)
              n231 = Divide(x=w404, y=i8 2) -> (x/y=w407:dbl)
              n232 = Less?(x=w395, y=0.5) -> (x < y?=w402:bool)
              n233 = Index Array(array=w396, index=0) -> (element=w399:string)
              n234 = Less?(x=w407, y=w403) -> (x < y?=w405:bool)
              n235 = And(x=w402, y=w405) -> (x .and. y?=w401:bool)
              n236 = Concatenate Strings(w399, "!" ("t")) -> (w397:string)
              n237 = Select(t=w397, s=w401, f="") -> (s? t:f=w408:string)
            }
          }
          n238 = case shown="1.." w372 {
            selector: w372 -> [_ w382]
            tunnel: [_ w380] -> w369
            tunnel: [_ w388] -> w370
            tunnel: [w374 w387] -> w366
            frame 0, Default {
              n239 = local read "case2"() -> (w375:i32)
              n240 = local read "var_2"() -> (w376:i8)
              n241 = Divide(x=w376, y=w375) -> (x/y=w374:dbl)
            }
            frame 1.. {
              n242 = local read "case2"() -> (w383:i32)
              n243 = local read "var_2"() -> (w389:i8)
              n244 = local read "Ex_Mod_IDs"() -> (w379:string[])
              n245 = Divide(x=w389, y=w383) -> (x/y=w387:dbl)
              n246 = Divide(x=w383, y=i8 2) -> (x/y=w384:dbl)
              n247 = Less?(x=w387, y=0.5) -> (x < y?=w381:bool)
              n248 = Less?(x=w384, y=w382) -> (x < y?=w386:bool)
              n249 = Index Array(array=w379, index=0) -> (element=w377:string)
              n250 = And(x=w381, y=w386) -> (x .and. y?=w380:bool)
              n251 = Select(t=w377, s=w380, f="") -> (s? t:f=w388:string)
            }
          }
          n252 = Not Exclusive Or(1:w369, 2:w368) -> (0:w362:bool)
          n253 = Concatenate Strings(w371, w370) -> (w361:string)
          n254 = Select(t="", s=w362, f=w361) -> (s? t:f=w359:string)
          n255 = Compound Arithmetic op=ADD(w367, w366) -> (w364:dbl)
          n256 = Divide(x=w364, y=2.0) -> (x/y=w363:dbl)
        }
      }
      n257 = local write "Boolean  Expression"(w214) -> ()
      n258 = Multiply(x=w212, y=100.0) -> (x*y=w209:dbl)
      n259 = Subtract(x=100.0 ("y"), y=w209) -> (x-y=w206:dbl)
      n260 = Number To Fractional String(number=w206, precision (6)=i16 2) -> (F-format string=w207:string)  [unwired: 2 in]
      n261 = case shown="Default" w207 {
        selector: w207 -> [w217 _]
        tunnel: [w216 "All input combinations are not applied correctly!" ("% fitness")] -> w205
        frame Default {
          n262 = local read "Input Status"() -> (w215:bool)
          n263 = case shown="True" w215 {
            tunnel: w217 -> [w222 _]
            tunnel: [w221 "All input combinations are not applied correctly!" ("% fitness")] -> w216
            frame False {
              n264 = property on="% fitness" class="Str"("Text.TextColor"=u32 2846208) -> ()  [unwired: 2 in, 2 out]
              n265 = property on="% fitness" class="Str"("Text.FontSize"=u32 25 ("Text.Font:Size")) -> ()  [unwired: 2 in, 2 out]
              n266 = Concatenate Strings("Fitness = ", w222, " %" ("string")) -> (w221:string)
            }
            frame True {
              n267 = property on="% fitness" class="Str"("Text.TextColor"=u32 15670016) -> ()  [unwired: 2 in, 2 out]
              n268 = property on="% fitness" class="Str"("Text.FontSize"=u32 17 ("Text.Font:Size")) -> ()  [unwired: 2 in, 2 out]
            }
          }
        }
        frame "NaN" {
          n269 = property on="% fitness" class="Str"("Text.TextColor"=u32 15670016) -> ()  [unwired: 2 in, 2 out]
          n270 = property on="% fitness" class="Str"("Text.FontSize"=u32 17 ("Text.Font:Size")) -> ()  [unwired: 2 in, 2 out]
        }
      }
      n271 = local write "% fitness"(w205) -> ()
    }
    frame #6 {
      # "Remove Empty strings and replace it with the previous expressions"
      n272 = local read "Boolean  Expression"() -> (w422:string)
      n273 = disable-structure shown="Enabled" {
        frame Enabled {
          n274 = while {
            tunnel: ["Close"] -> w440
            stop <- "Close" stop-if-true
            n275 = Wait Until Next ms Multiple(millisecond multiple=u32 1) -> ()  [unwired: 1 out]
          }
          "Close 2" <- w440
          n276 = Not(x=w440) -> (.not. x?=w439:bool)
          n277 = property class="VI"("Front Panel Window:Open"=w439) -> ()  [unwired: 2 in, 2 out]
        }
        frame Disabled {
        }
      }
      n278 = local read "Ex_Mod_IDs"() -> (w423:string[])
      n279 = call "2-input AND.vi"("Obtained Expression"=w422, "Input List"=w423) -> ("AND ?"=w428:bool, "Logic Exp"=w429:string)  [unwired: 7 in, 1 out]
      n280 = call "2-input NAND.vi"("Obtained Expression"=w422, "Input List"=w423) -> ("NAND ?"=w438:bool, "Logic Exp"=w433:string)  [unwired: 7 in, 1 out]
      n281 = call "2-input OR.vi"("Obtained Expression"=w422, "Input List"=w423) -> ("OR ?"=w437:bool, "Logic Exp"=w434:string)  [unwired: 7 in, 1 out]
      n282 = call "2-input NOR.vi"("Obtained Expression"=w422, "Input List"=w423) -> ("Nand ?"=w436:bool, "Logic Exp"=w435:string)  [unwired: 7 in, 1 out]
      n283 = call "2-input NOT.vi"("Obtained Expression"=w422, "Input List"=w423) -> ("NOT ?"=w424:bool, "Logic Exp"=w425:string)  [unwired: 7 in, 1 out]
      n284 = local read "Boolean  Expression"() -> (w413:string)
      n285 = Select(t=w429, s=w428, f="") -> (s? t:f=w427:string)
      n286 = Select(t=w433, s=w438, f="") -> (s? t:f=w430:string)
      n287 = Select(t=w434, s=w437, f="") -> (s? t:f=w431:string)
      n288 = Select(t=w435, s=w436, f="") -> (s? t:f=w432:string)
      n289 = Select(t=w425, s=w424, f="") -> (s? t:f=w421:string)
      n290 = Concatenate Strings(w427, w430, w431, w432, w421) -> (w412:string)
      n291 = Equal?(x=w412, y="") -> (x = y?=w415:bool)
      n292 = Select(t=w413, s=w415, f=w412) -> (s? t:f=w414:string)
      n293 = local write "Boolean  Expression"(w414) -> ()
    }
  }
  n294 = local write "C1_Ar"(w26) -> ()
  n295 = local write "C2_Ar"(w26) -> ()
  n296 = local write "C3_Ar"(w26) -> ()
  n297 = local write "C4_Ar"(w26) -> ()
  n298 = local write "Thresh Val"(i32[] [] ("Array")) -> ()
  n299 = local write "Input Status"(FALSE ("Input Status")) -> ()
  "Digital Data" <- bool[][] [] ("Dig. Data to Process")
  "C1" <- w21
  "C2" <- w21
  "C3" <- w21
  "C4" <- w21
  "case1" <- w22
  "case2" <- w22
  "case3" <- w22
  "case4" <- w22
  "var_1" <- w22
  "var_2" <- w22
  "var_3" <- w22
  "var_4" <- w22
  "Cs1_1s" <- w22
  "Cs2_1s" <- w22
  "Cs3_1s" <- w22
  "Cs4_1s" <- w22
  "Boolean  Expression" <- ""
  "Analog Data" <- dbl[][] [] ("Data to process")
  "Simulation Data" <- string[][] [] ("Table Control")
  "Row header" <- string[] [] ("Row header 2")
  "% fitness" <- ""
